vi "Handle setConfiguration.vi"(8 "error in (no error)":errorcluster, 10 "setConfiguration":variant, 11 "Inst.Krohn-Hite-7008 in":refnum<class "Inst.Krohn-Hite-7008.lvclass">) -> (0 "error out":errorcluster, 3 "Inst.Krohn-Hite-7008 out":refnum<class "Inst.Krohn-Hite-7008.lvclass">)   [LabVIEW 2019, in "Inst.Krohn-Hite-7008.lvclass"]
uses:
  Inst.Krohn-Hite-7008.lvclass
  Inst.Krohn-Hite-7008.lvclass/Inst.Krohn-Hite-7008.ctl
  45e4b271-6884-462c-ad3a-d505ab08eb62.vi
  45e4b271-6884-462c-ad3a-d505ab08eb62.vi/cc912182-6aba-4858-9323-8e0d5cc13759.vi
  45e4b271-6884-462c-ad3a-d505ab08eb62.vi/f455c486-0eba-40a4-bbf0-29ee5eb23354.vi
  <vilib>/Utility/Data Type/Get Type Information.vi
  <vilib>/JDP Science/JSONtext/JSON text to Variant.vi
  <vilib>/JDP Science/JSONtext/LVClass Serializer/JSONtext LVClass Serializer.lvclass
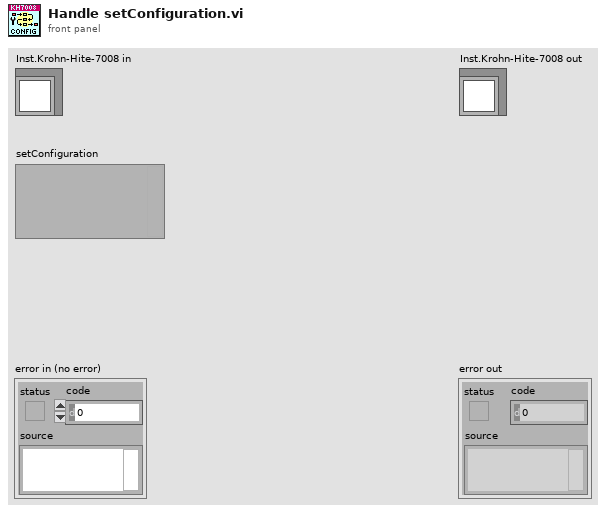
[diagram p1: front panel]
types:
  T1 = typedef "Inst.Krohn-Hite-7008.lvclass/Inst.Krohn-Hite-7008.Configuration--Cluster.ctl" = cluster{"Visa Ref":refnum<visa-resource-name>, "Serial No":string}
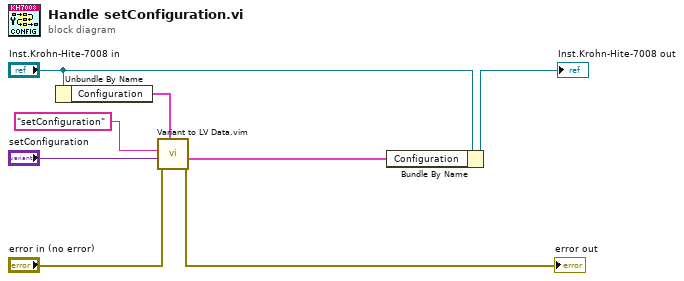
[diagram p0: block diagram]
diagram:
  n1 = Unbundle By Name("Inst.Krohn-Hite-7008 in") -> ("Configuration"=w7:T1)
  n2 = call "Variant to LV Data.vim"("type"=w7, "error in (no error)"="error in (no error)", "JSON Data in"="setConfiguration", "Command"="setConfiguration") -> ("error out"=→"error out":errorcluster, "Data out"=w1:T1)  [unwired: 4 in, 2 out]
  n3 = Bundle By Name(cluster="Inst.Krohn-Hite-7008 in", "Configuration"=w1) -> (→"Inst.Krohn-Hite-7008 out":refnum<class "Inst.Krohn-Hite-7008.lvclass">)
